vi "Write Instruments.vi"(8 "error in (no error)":errorcluster, 10 "Instruments":refnum<class "Generic Item.lvclass">[](array[class]), 11 "Category in":refnum<class "Category.lvclass">) -> (0 "error out":errorcluster, 3 "Category out":refnum<class "Category.lvclass">)   [LabVIEW 2015, in "Category Library.lvlib" / "Category.lvclass"]
uses:
  Category.lvclass
  Generic Item/Generic Item.lvclass
  Category.lvclass/Category.ctl
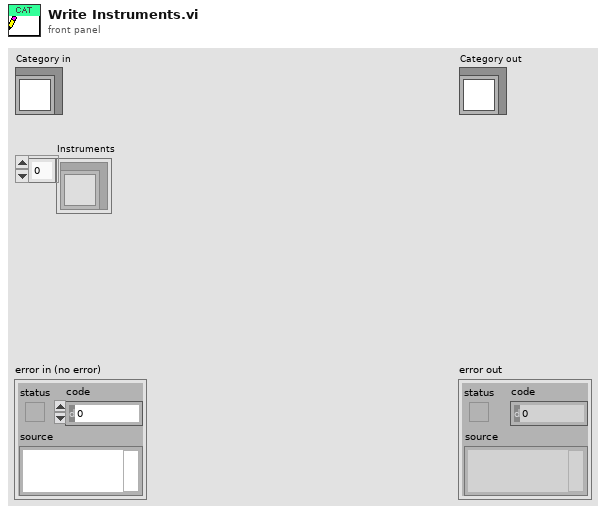
[diagram p1: front panel]
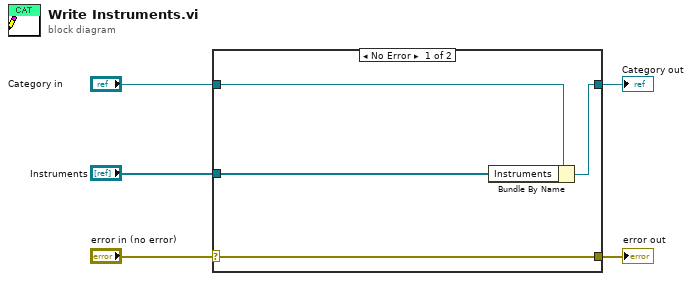
[diagram p0: block diagram]
diagram:
  n1 = case shown="No Error" "error in (no error)" {
    selector: "error in (no error)" -> [w9 w10]
    tunnel: [w9 w10] -> w4
    tunnel: [w7 w11] -> w2
    tunnel: "Category in" -> [w8 w11]
    tunnel: "Instruments" -> [w6 _]
    frame No Error {
      n2 = Bundle By Name(cluster=w8, "Instruments"=w6) -> (w7:refnum<class "Category.lvclass">)
    }
    frame Error {
    }
  }
  "error out" <- w4
  "Category out" <- w2
